vi "例5.8   利用循环结构生成数组.vi"() -> ()   [LabVIEW 2017]
panel:
  out "输出数组":i32[](array[numeric])
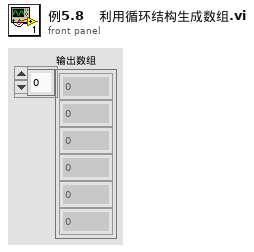
[diagram p1: front panel]
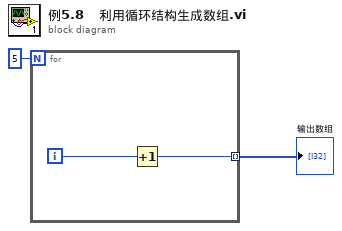
[diagram p0: block diagram]
diagram:
  n1 = for {
    N: 5 -> [_]
    tunnel: [w3] -> w1 mode=indexing
    i -> [w4]
    n2 = Increment(x=w4) -> (x+1=w3:i32)
  }
  "输出数组" <- w1
